vi "Test the VNA class sub class.vi"() -> ()   [LabVIEW 2020, in "Vector Network Analyzer.lvclass"]
uses:
  Vector Network Analyzer.lvclass
  Controls/Sparameter cluster.ctl
  VNA-ZNB/VNA-ZNB.lvclass
  Controls/S parm format enum.ctl
  C:/Sandbox/Git_Sandbox/WiSpry Test Framework source code (LV20)/WiSpry Test Framework/Instruments/Instrument.lvclass
  VNA-Ag87xx/VNA-Ag87xx.lvclass
  VNA-ENA/VNA-ENA.lvclass
  VNA-FieldFox/VNA-FieldFox.lvclass
  C:/Sandbox/Git_Sandbox/WiSpry Test Framework source code (LV20)/WiSpry Test Framework/Instruments/Vector Network Analyzer/Vector Network Analyzer.lvclass
  Instrument.lvclass/Instrument.ctl
  Instrument.lvclass
panel:
  out "S parameters":T1[](array[typedef])
  out "XY Graph":cluster{"Frequency":dbl[], "Data":dbl[]}(graph)
  out "Marker Data":dbl
  out "Marker Frequency":dbl
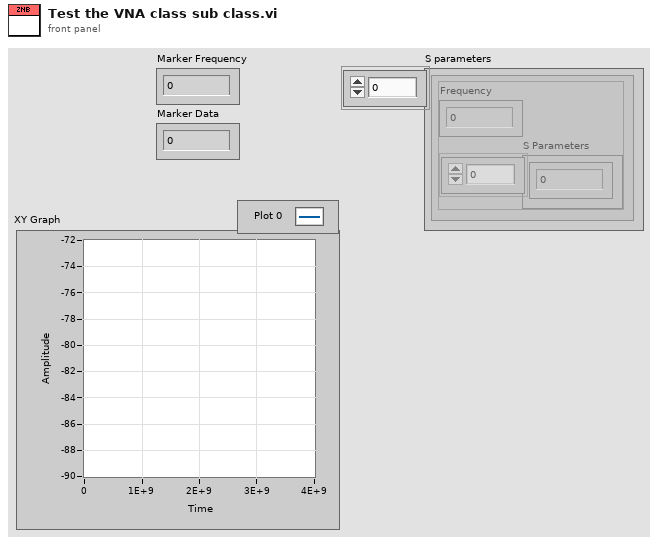
[diagram p1: front panel]
types:
  T1 = typedef "Vector Network Analyzer.lvclass/Sparameter cluster.ctl" = cluster{"Frequency":dbl, "S Parameters":cdb[]}
  T2 = typedef "Vector Network Analyzer.lvclass/S parm format enum.ctl" = enum16{"Mag dB", "Mag", "Phase", "Smith", "Real", "Imag", "Group Delay", "SWR"}
  T3 = enum16{"S11", "S21", "S31", "S41", "S22", "S12", "S32", "S42", "S33", "S13", "S23", "S43", "S44", "S14", "S24", "S34"}
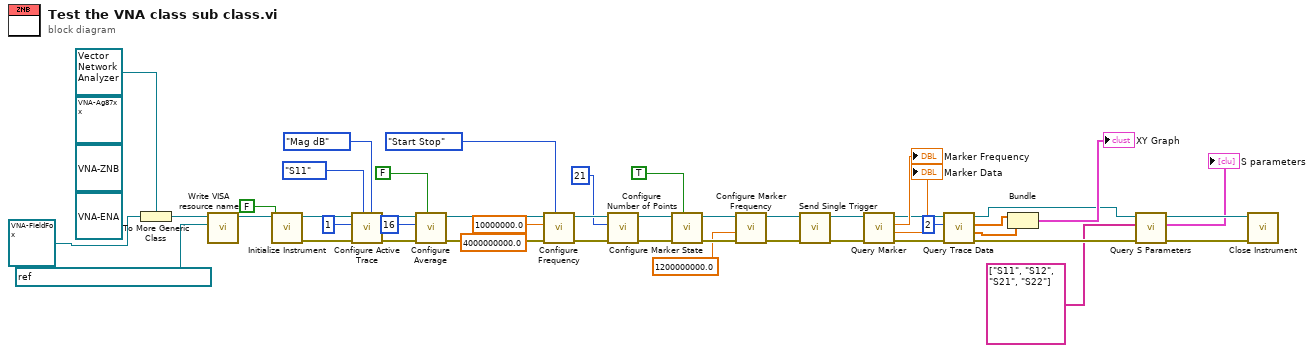
[diagram p0: block diagram]
diagram:
  (unwired) refnum<class "VNA-ENA.lvclass"> refnum ("VNA-ENA.lvclass")
  (unwired) refnum<class "VNA-Ag87xx.lvclass"> refnum ("VNA-Ag87xx.lvclass")
  (unwired) refnum<class "VNA-ZNB.lvclass"> refnum ("VNA-ZNB.lvclass")
  n1 = To More Generic Class(target class=refnum<class "Vector Network Analyzer.lvclass"> refnum ("Vector Network Analyzer.lvclass"), reference=refnum<class "VNA-FieldFox.lvclass"> refnum ("VNA-FieldFox.lvclass")) -> (generic class reference=w11:refnum<class "Vector Network Analyzer.lvclass">)
  n2 = call "Write VISA resource name.vi"("VISA resource name"=refnum<visa-resource-name> "TCPIP0::192.168.1.6::inst0::INSTR", "Instrument in"=w11) -> ("Instrument out"=w47:refnum<class "Vector Network Analyzer.lvclass">)  [unwired: 9 in]
  n3 = call-dynamic "Initialize Instrument.vi"("Reset"=FALSE, "Instrument in"=w47) -> ("error out"=w46:errorcluster, "Instrument out"=w45:refnum<class "Vector Network Analyzer.lvclass">)  [unwired: 8 in]
  n4 = call-dynamic "Configure Active Trace.vi"("Format"=S_parm_format_enum."Mag dB", "S parameter"=T3."S11", "error in (no error)"=w46, "Active Trace"=u8 1, "Vector Network Analyzer in"=w45) -> ("error out"=w41:errorcluster, "Vector Network Analyzer out"=w40:refnum<class "Vector Network Analyzer.lvclass">)  [unwired: 5 in]
  n5 = call-dynamic "Configure Average.vi"("Average On"=FALSE, "error in (no error)"=w41, "Number of Averages"=16, "Vector Network Analyzer in"=w40) -> ("error out"=w37:errorcluster, "Vector Network Analyzer out"=w36:refnum<class "Vector Network Analyzer.lvclass">)  [unwired: 6 in]
  n6 = call-dynamic "Configure Frequency.vi"("Mode"=enum16{"Center Span", "Start Stop"}."Start Stop", "error in (no error)"=w37, "Span/Stop Frequency"=4000000000.0, "Center/Start Frequency"=10000000.0, "Vector Network Analyzer in"=w36) -> ("error out"=w32:errorcluster, "Vector Network Analyzer out"=w31:refnum<class "Vector Network Analyzer.lvclass">)  [unwired: 5 in]
  n7 = call-dynamic "Configure Number of Points.vi"("error in (no error)"=w32, "Number of Point"=21, "Vector Network Analyzer in"=w31) -> ("error out"=w29:errorcluster, "Vector Network Analyzer out"=w28:refnum<class "Vector Network Analyzer.lvclass">)  [unwired: 7 in]
  n8 = call-dynamic "Configure Marker State.vi"("Marker On"=TRUE, "error in (no error)"=w29, "Vector Network Analyzer in"=w28) -> ("error out"=w26:errorcluster, "Vector Network Analyzer out"=w25:refnum<class "Vector Network Analyzer.lvclass">)  [unwired: 7 in]
  n9 = call-dynamic "Configure Marker Frequency.vi"("error in (no error)"=w26, "Marker Frequency"=1200000000.0, "Vector Network Analyzer in"=w25) -> ("error out"=w23:errorcluster, "Vector Network Analyzer out"=w22:refnum<class "Vector Network Analyzer.lvclass">)  [unwired: 7 in]
  n10 = call-dynamic "Send Single Trigger.vi"("error in (no error)"=w23, "Vector Network Analyzer in"=w22) -> ("error out"=w21:errorcluster, "Vector Network Analyzer out"=w20:refnum<class "Vector Network Analyzer.lvclass">)  [unwired: 8 in]
  n11 = call-dynamic "Query Marker.vi"("error in (no error)"=w21, "Vector Network Analyzer in"=w20) -> ("error out"=w17:errorcluster, "Data"=→"Marker Data":dbl, "Frequency"=→"Marker Frequency":dbl, "Vector Network Analyzer out"=w16:refnum<class "Vector Network Analyzer.lvclass">)  [unwired: 6 in]
  n12 = call-dynamic "Query Trace Data.vi"("error in (no error)"=w17, "Trace Number"=u8 2, "Vector Network Analyzer in"=w16) -> ("error out"=w9:errorcluster, "Data"=w14:dbl[], "Frequency"=w15:dbl[], "Vector Network Analyzer out"=w8:refnum<class "Vector Network Analyzer.lvclass">)  [unwired: 5 in]
  n13 = Bundle("Frequency"=w15, "Data"=w14) -> (→"XY Graph":cluster{"Frequency":dbl[], "Data":dbl[]})  [unwired: 1 in]
  n14 = call-dynamic "Query S Parameters.vi"("error in (no error)"=w9, "Sparameters (string)"=string[] ["S11", "S12", "S21", "S22"], "Vector Network Analyzer in"=w8) -> ("error out"=w6:errorcluster, "S parameters"=→"S parameters":T1[], "Vector Network Analyzer out"=w7:refnum<class "Vector Network Analyzer.lvclass">)  [unwired: 6 in]
  n15 = call-dynamic "Close Instrument.vi"("error in (no error)"=w6, "Instrument in"=w7) -> ()  [unwired: 8 in, 2 out]
